vi "RPM to Radians per Second.vi"   [LabVIEW 2020, in "NI_AngleConversion.lvlib"]
doc: "Converts data from revolutions per minute (RPM) to radians per second."
uses:
  <vilib>/Analysis/NI_AngleConversion.lvlib
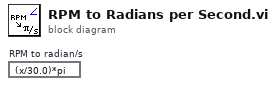
[diagram p0: block diagram]
diagram:
  n1 = expression code="(x/30.0)*pi" "RPM to radian/s"() -> ()  [unwired: 1 in, 1 out]
